vi "Do.vi"(8 "error in (no error)":errorcluster, 10 "Actor in":refnum<class "Actor.lvclass">, 11 "Go To Work Msg":refnum<class "Go To Work Msg.lvclass">) -> (0 "error out":errorcluster, 2 "Actor out":refnum<class "Actor.lvclass">)   [LabVIEW 2024, in "Test States.lvlib" / "Go To Work Msg.lvclass"]
doc: "This VI delivers the message to the actor by calling the appropriate method(s) on the actor."
uses:
  Go To Work Msg.lvclass
  <vilib>/ActorFramework/Actor/Actor.lvclass
  Test State/Test State.lvclass
  C:/Program Files/National Instruments/LabVIEW 2024/vi.lib/ActorFramework/Actor/Actor.lvclass
  Go To Work Msg.lvclass/Go To Work Msg.ctl
  C:/Program Files/National Instruments/LabVIEW 2024/vi.lib/ni/Actors/State Actor/State Actor/State Actor.lvclass
  C:/Users/burakkorkmaz/Desktop/PROJE/actor-state-machine/Test States/Test State/Test State.lvclass
  <vilib>/ni/Actors/State Actor/State Actor/State Actor.lvclass
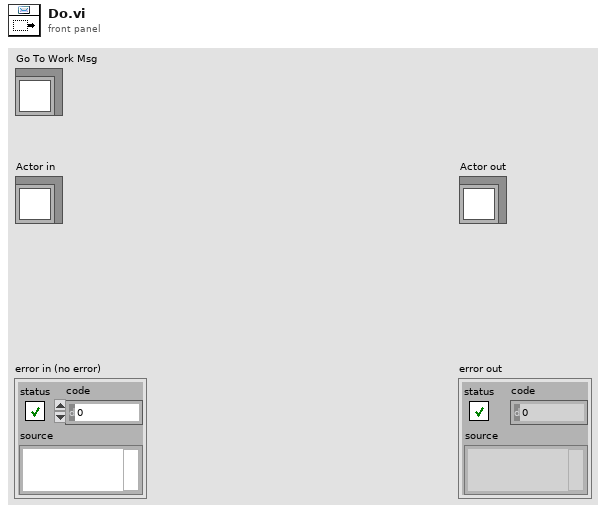
[diagram p1: front panel]
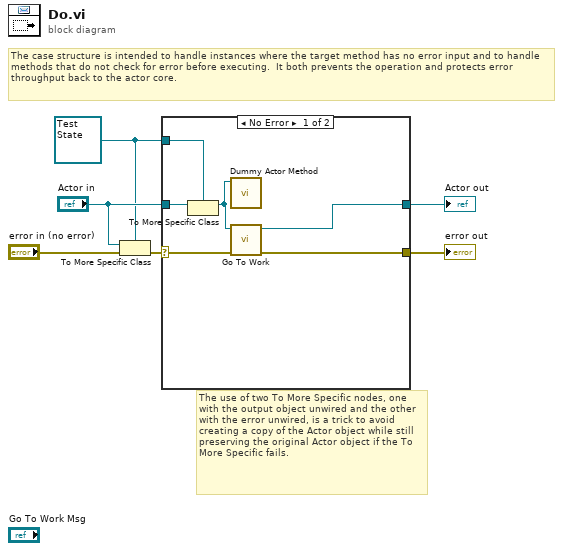
[diagram p0: block diagram]
diagram:
  w2 = refnum<class "Test State.lvclass"> refnum ("Actor in")
  # "The use of two To More Specific nodes, one with the output object unwired and the other with the error unwired, is a trick to avoid creating a copy of the Actor object while still preserving the original Actor object if the To More Specific fails."
  # "The case structure is intended to handle instances where the target method has no error input and to handle methods that do not check for error before executing.  It both prevents the operation and protects error throughput back to the actor core."
  n1 = To More Specific Class(target class=w2, reference="Actor in", error in="error in (no error)") -> (error out=w1:errorcluster)  [unwired: 1 out]
  n2 = case shown="No Error" w1 {
    selector: w1 -> [w12 w14]
    tunnel: [w9 w14] -> w6
    tunnel: [w7 w13] -> w5
    tunnel: "Actor in" -> [w8 w13]
    tunnel: w2 -> [w10 _]
    frame No Error {
      n3 = To More Specific Class(target class=w10, reference=w8) -> (specific class reference=w11:refnum<class "Test State.lvclass">)  [unwired: 1 in, 1 out]
      n4 = call <resource>:"Dummy Actor Method.vi"("Actor in"=w11) -> ()  [unwired: 9 in, 2 out]
      n5 = call-dynamic "Go To Work.vi"("error in (no error)"=w12, "Test State in"=w11) -> ("error out"=w9:errorcluster, "State Actor.lvclass"=w7:refnum<class "State Actor.lvclass">)  [unwired: 8 in]
    }
    frame Error {
      # "If type check fails, pass the original object out again."
    }
  }
  "error out" <- w6
  "Actor out" <- w5
